vi "Find Children of Node.vi"(8 "error in":errorcluster, 10 "Node":T2, 11 "Fast Tree in":refnum<class "Fast Tree.lvclass">) -> (0 "error out":errorcluster, 2 "Children":T1(array[cluster]), 3 "Fast Tree out":refnum<class "Fast Tree.lvclass">)   [LabVIEW 2019, in "Fast Tree.lvclass"]
uses:
  Fast Tree.lvclass
  Fast Tree.lvclass/Fast Tree.ctl
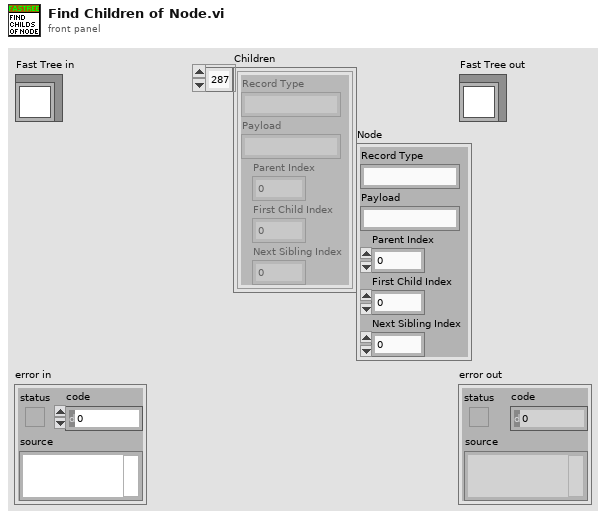
[diagram p1: front panel]
types:
  T1 = cluster{"Record Type":string, "Payload":string, "Parent Index":i32, "First Child Index":i32, "Next Sibling Index":i32}[]
  T2 = cluster{"Record Type":string, "Payload":string, "Parent Index":i32, "First Child Index":i32, "Next Sibling Index":i32}
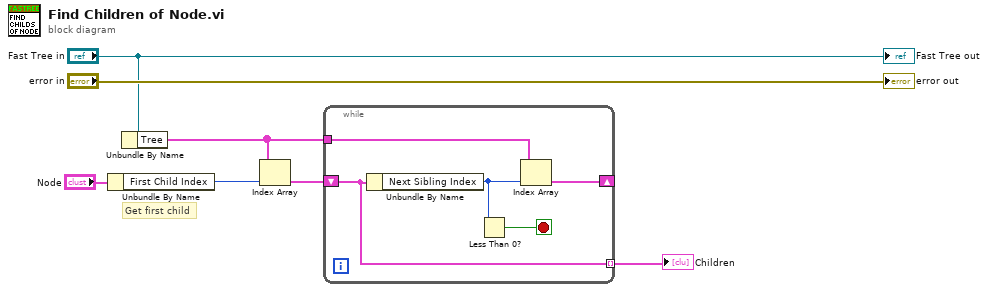
[diagram p0: block diagram]
diagram:
  # "Get first child"
  n1 = Unbundle By Name("Node") -> ("First Child Index"=w1:i32)
  n2 = Unbundle By Name("Fast Tree in") -> ("Tree"=w3:T1)
  n3 = Index Array(array=w3, index=w1) -> (element=w4:T2)
  n4 = while {
    tunnel: [w11] -> w2 mode=indexing
    tunnel: w3 -> [w10]
    shift-right: [w9] -> _
    shift-left: w4 -> [w11]
    stop <- w12 stop-if-true
    n5 = Unbundle By Name(w11) -> ("Next Sibling Index"=w8:i32)
    n6 = Less Than 0?(x=w8) -> (x < 0?=w12:bool)
    n7 = Index Array(array=w10, index=w8) -> (element=w9:T2)
  }
  "Children" <- w2
  "error out" <- "error in"
  "Fast Tree out" <- "Fast Tree in"
